vi "PDF Protokoll EPA1065_InterferenceVerification.vi"(8 "error in (no error)":errorcluster caption="Fehler (Eingang, kein Fehler)") -> (0 "error out":errorcluster caption="Fehler (Ausgang)")   [LabVIEW 2020, in "EPA 1065.lvlib" / "Interference verificaton 1065-366.lvlib"]
uses:
  Interference verificaton 1065-366.lvlib
  Visualisierungs Elemente/String - Ausgabefeld.ctl
  ResultTable.ctl
  Sprachverwaltung/FGV Aktion Tabelle zerlegen.ctl
  <vilib>/Utility/miscctls.llb/LVRowAndColumnTypeDef.ctl
  Aktion FGV Interference.ctl
  Seiten/FT-IR/FGV FT-IR Aktionen.ctl
  Aktion Index uebersetzten.ctl
  Seiten/System Einstellungen V2/Aktioen FGV System Konstanten.ctl
  <vilib>/Utility/miscctls.llb/LVPrintingMarginsTypeDef.ctl
  Allgemein/allgemeine Sub-VIs.lvlib
  Seiten/FT-IR/Span/Spanfaktor.lvlib
  Seiten/FT-IR/FT-IR.lvlib
  Sprachverwaltung/Sprachverwaltung.lvlib
  Seiten/System Einstellungen V2/System Einstellungen V2.lvlib
panel:
  out "Grenze in ppm:":sgl=2.0 caption="Limit in ppm:" min=0 format="%#.6g"
  out "[%]":sgl=2.0 caption="Limit:" min=0 format="%#.6g"
  out "LIN Ausgabetabelle":T1
  out "[%]":sgl=120.0 caption="Interference:" min=0 format="%#.6g"
  out "Konzentration Komponente":sgl=120.0 caption="Concentration:" min=0
  out "Komponente:":T2 caption="ppm"
  out "max. Flow Weighted Mean:":T2 caption="%"
  out "Konzentration FlowWeightedMean":sgl=120.0 caption="Concentration:" min=0 format="%#.2f"
  out "Tabelle 3":string[][](table)
  out "Tabelle":string[][](table)
  # "Interference Verification - EPA § 1065.366"
  # "Result"
  # "Analysis"
  # "Interference for Component:"
  # "Expected Flow weighted mean:"
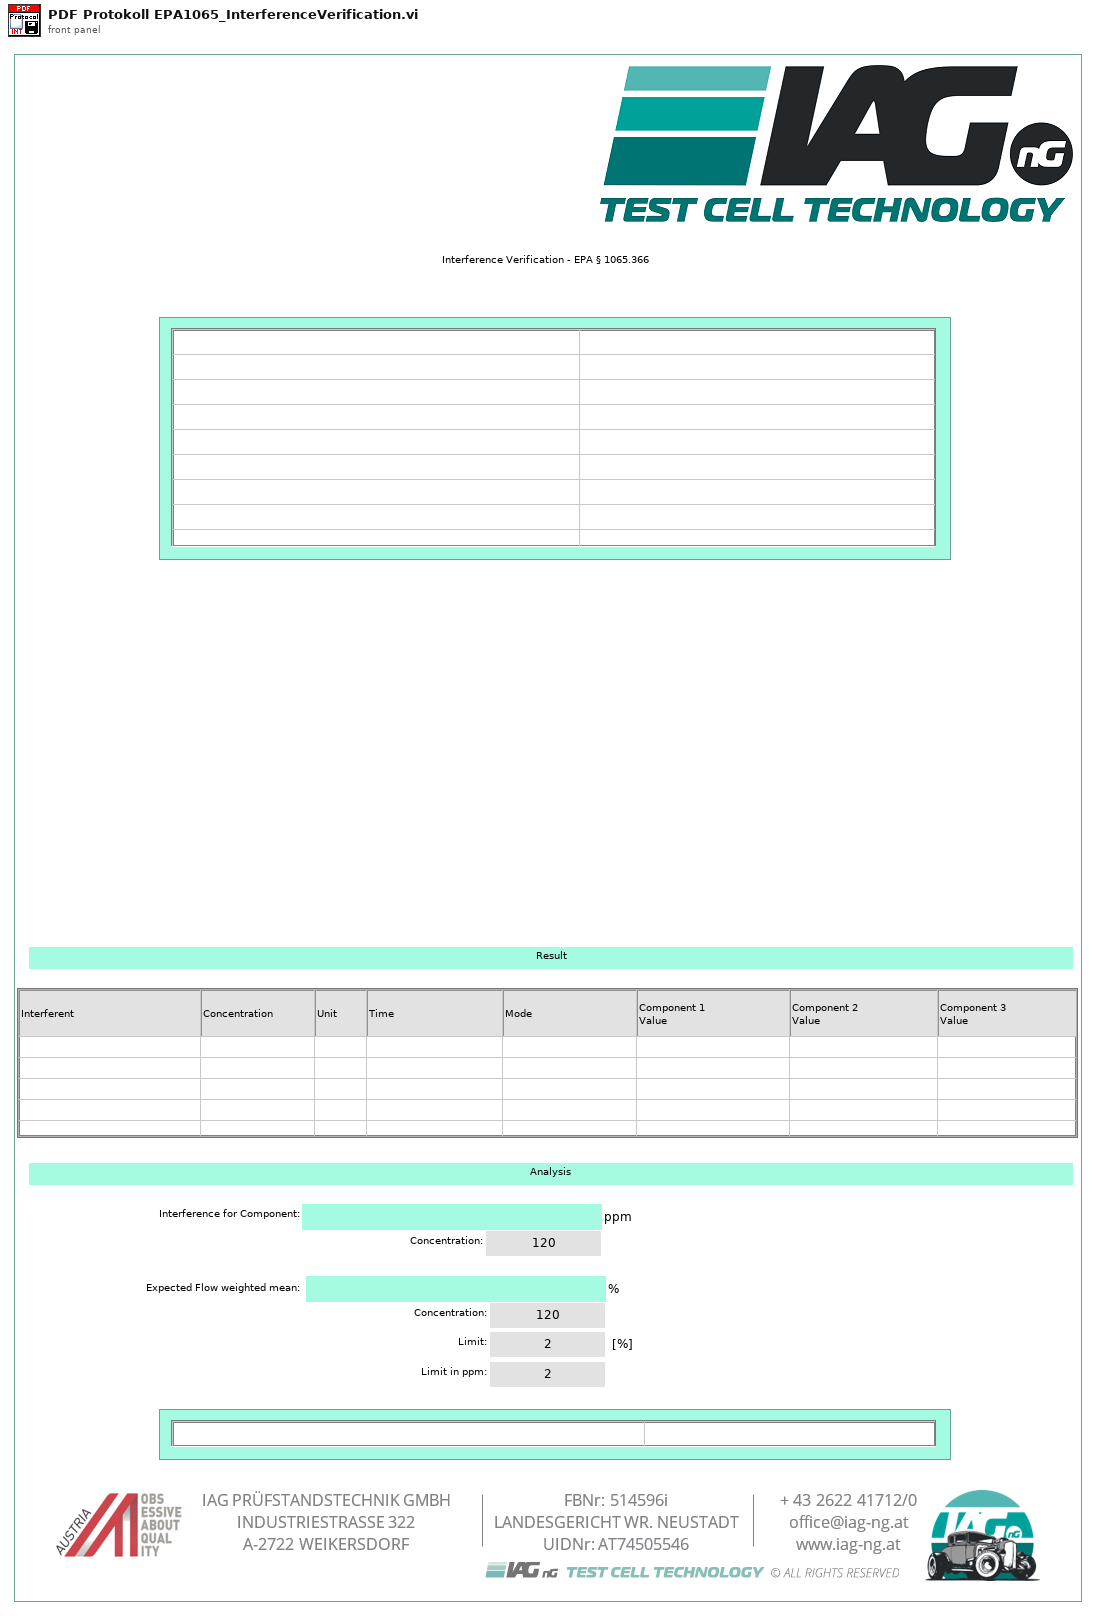
[diagram p1: front panel]
types:
  T1 = typedef "EPA 1065.lvlib/Interference verificaton 1065-366.lvlib/ResultTable.ctl" = string[][]
  T2 = typedef "String - Ausgabefeld.ctl" = string
  T3 = typedef "Sprachverwaltung.lvlib/FGV Aktion Tabelle zerlegen.ctl" = enum16{"laden", "vereinzeln", "speichern"}
  T4 = typedef "System Einstellungen V2.lvlib/Aktioen FGV System Konstanten.ctl" = enum16{"lesen", "laden", "speichern", "Sprache"}
  T5 = typedef "EPA 1065.lvlib/Interference verificaton 1065-366.lvlib/Aktion Index uebersetzten.ctl" = enum16{"lesen", "schreiben", "auswerten"}
  T6 = typedef "FT-IR.lvlib/FGV FT-IR Aktionen.ctl" = enum16{"lesen", "NOG setzen", "NOS setzen", "Initialisieren", "speichern", "ALLES setzen", "FT-IR Spektrum loggen", "Komm Stoppen", "Spektrum LogKonfig"}
  T7 = typedef "EPA 1065.lvlib/Interference verificaton 1065-366.lvlib/Aktion FGV Interference.ctl" = enum16{"Lesen", "TestKonfig", "TestSetting", "Einheiten", "Ergebnis", "Laden", "Tabelle", "Speichern", "löschen"}
  T8 = typedef "LVRowAndColumnTypeDef.ctl" = cluster{"Row":i32, "Column":i32}
  T9 = typedef "LVPrintingMarginsTypeDef.ctl" = cluster{"Top":sgl, "Left":sgl, "Bottom":sgl, "Right":sgl, "Measurement System":enum8{"Inches", "cm"}}
  T10 = enum32{"Portrait", "Landscape", "Rotated Portrait", "Rotated Landscape"}
  T11 = typedef "EPA 1065.lvlib/Interference verificaton 1065-366.lvlib/TestSetting.ctl" = cluster{"Bearbeiter:":string, "Pfad:":path, "Textname:":string, "Analysator":T12}
  T12 = typedef "System Einstellungen V2.lvlib/Analysatoren.ctl" = string
  T13 = typedef "EPA 1065.lvlib/Interference verificaton 1065-366.lvlib/TestKonfig.ctl" = cluster{"CH4:":u16, "Ethane:":u16, "NMHC:":u16, "NMNEHC:":u16, "Komp 1 aktiv:":bool, "Komp 2 aktiv:":bool, "Komp 3 aktiv:":bool, "Komp 4 aktiv:":bool, "Modus":T14, "CG Aufschaltzeit:":dbl, "Interferent 1: CO2":u16, "Interferent 2: H2O":u16, "Interferent 3: CH4":u16, "Interferent 4: C2H6 / C3H8":u16, "Gasflaschen Nr.:":string, "Gasflaschen Nr.: 3":string, "Gasflaschen Nr.: 4":string, "Inter 1 aktiv":bool, "Inter 2 aktiv":bool, "Inter 3 aktiv":bool, "Inter 4 aktiv":bool, "Accuracy":string, "Accuracy 3":string, "Accuracy 4":string, "Konzentration 1:":dbl, "Konzentration 2:":dbl, "Konzentration 3:":dbl, "Konzentration 4:":dbl, "Flow weighted mean 1:":dbl, "Flow weighted mean 2:":dbl, "Flow weighted mean 3:":dbl, "Flow weighted mean 4:":dbl}
  T14 = typedef "EPA 1065.lvlib/Interference verificaton 1065-366.lvlib/Modus.ctl" = u16
  T15 = typedef "EPA 1065.lvlib/Interference verificaton 1065-366.lvlib/Komponenten.ctl" = cluster{"Komponente":T2, "Komponente Index":i32, "Komponente 2":T2, "Komponente Index 2":i32, "Komponente 3":T2, "Komponente Index 3":i32, "Komponente 4":T2, "Komponente Index 4":i32, "Interferent 1":T2, "Interferent Index":i32, "Interferent 2":T2, "Interferent 2 Index":i32, "Interferent 3":T2, "Interferent 3 Index":i32, "Interferent 4":T2, "Interferent 4 Index":i32}
  T16 = cluster{"Modell":string, "ProjektNummer":string, "Software Version":string, "Seriennummer":string}
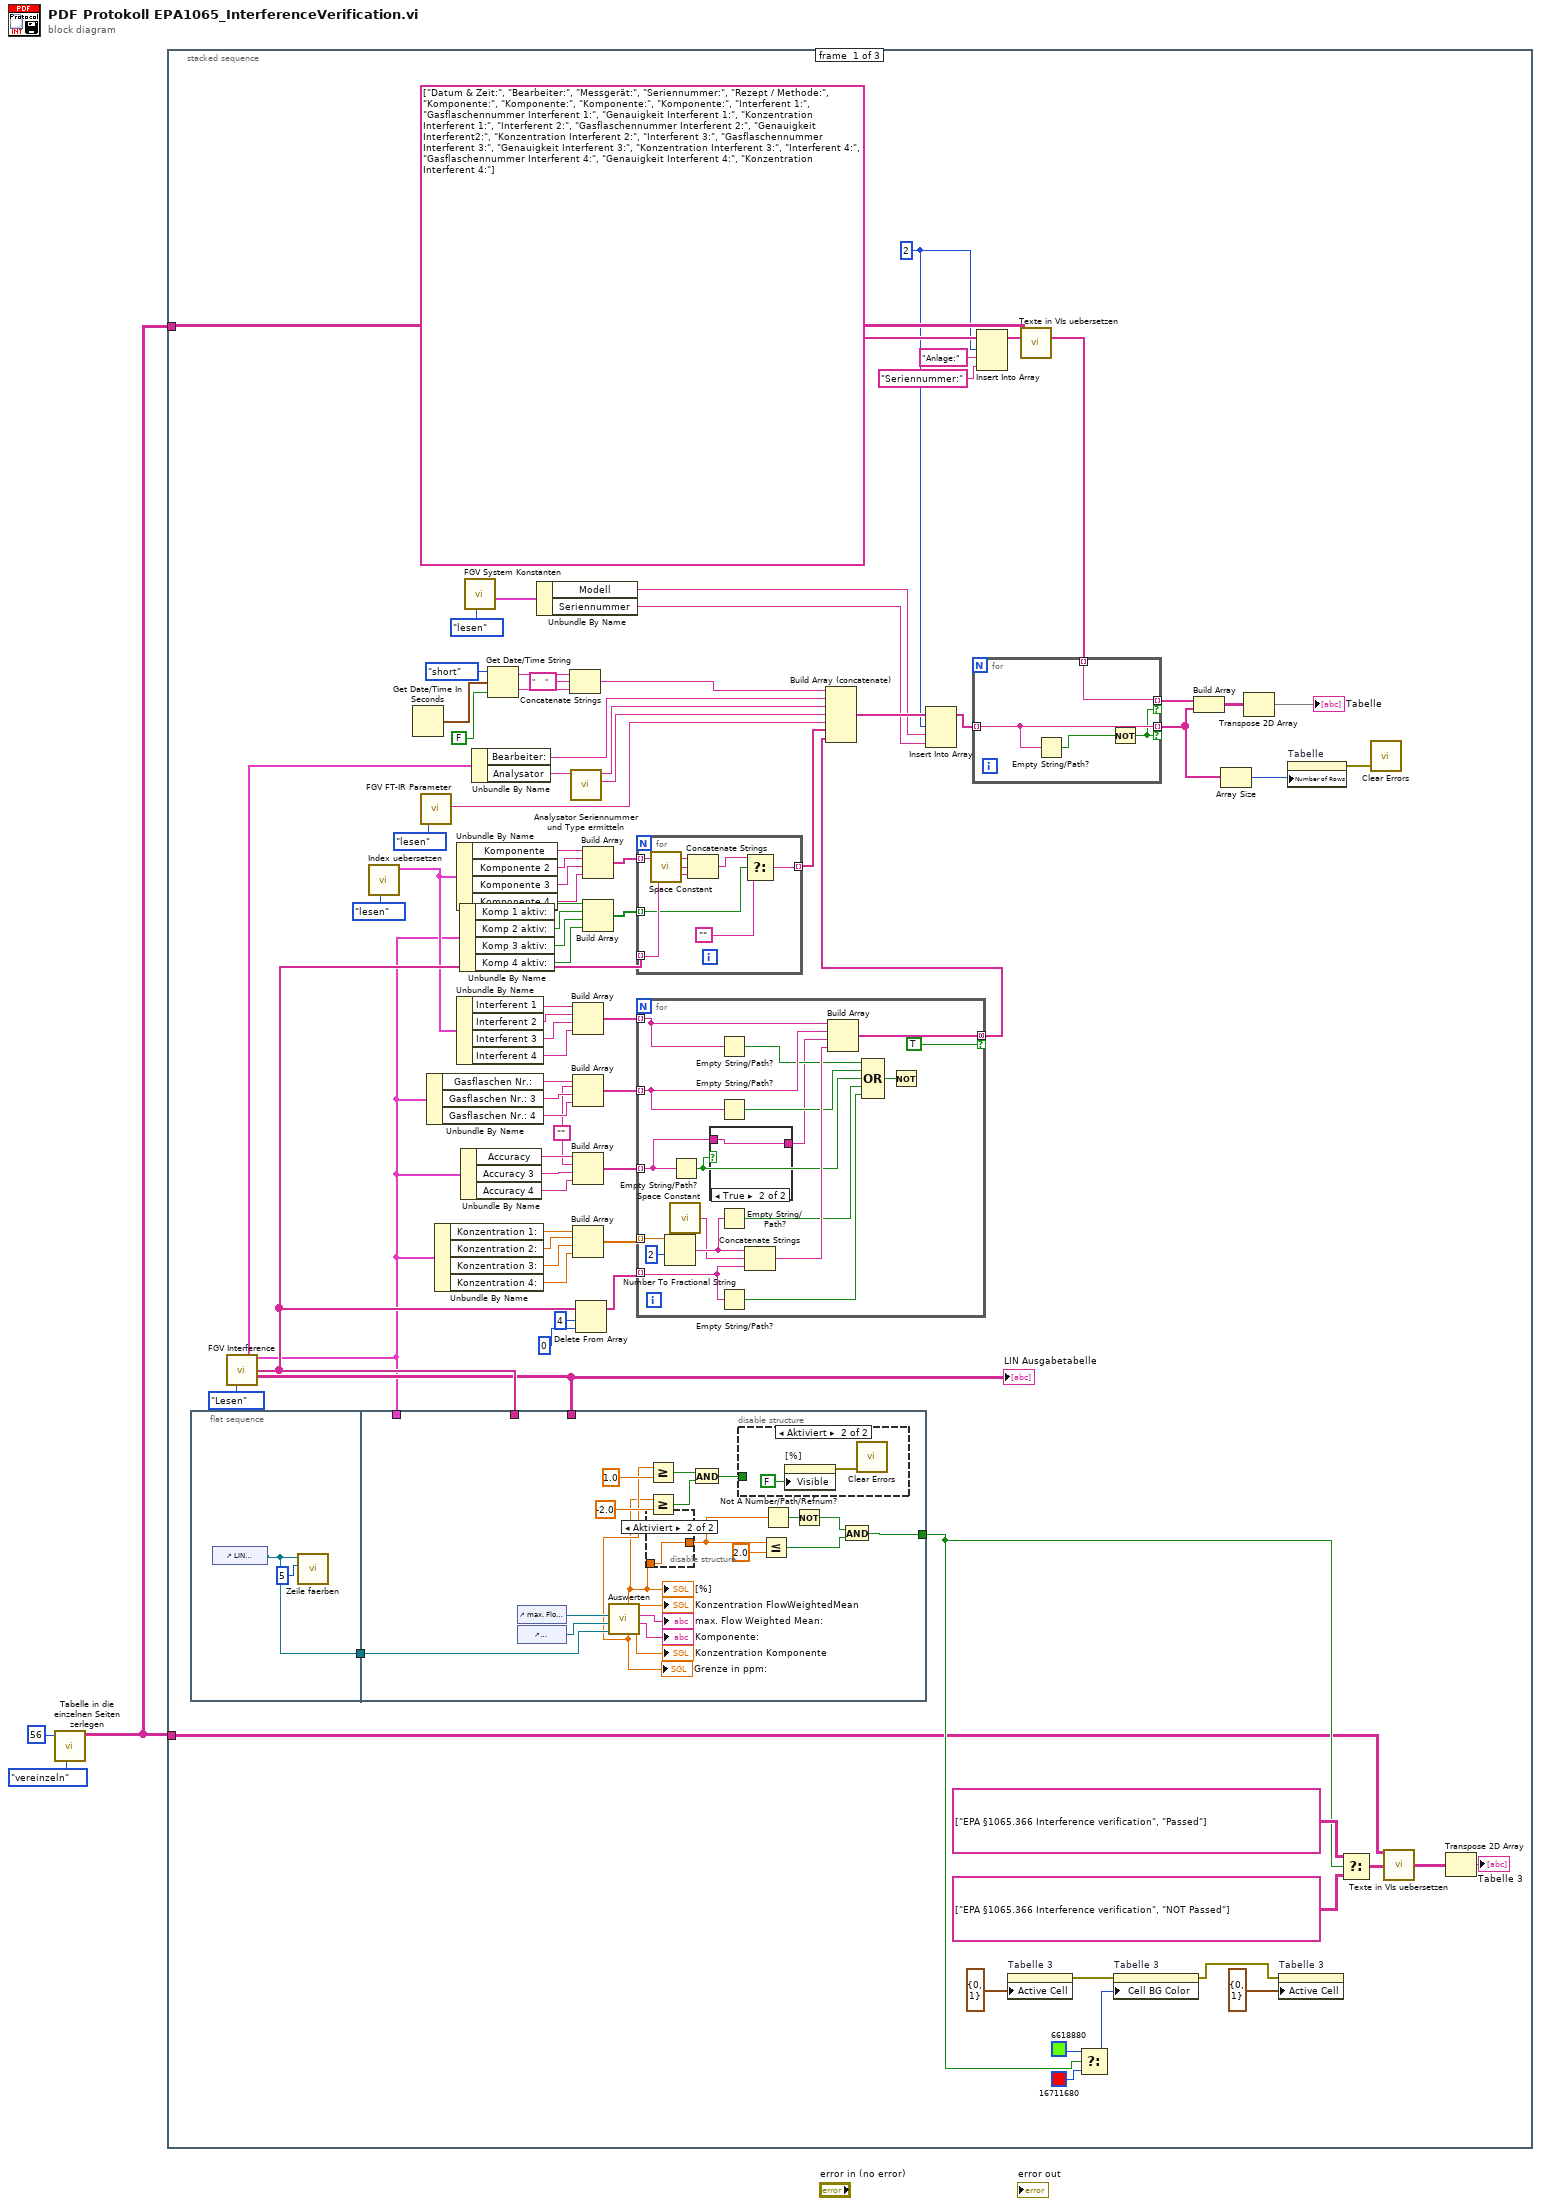
[diagram p0: block diagram]
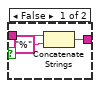
[diagram p2: hidden frame]
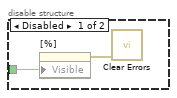
[diagram p3: hidden frame]
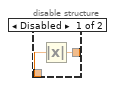
[diagram p4: hidden frame]
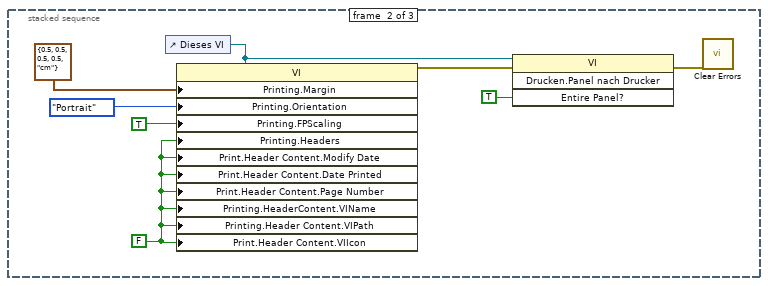
[diagram p5: hidden frame]
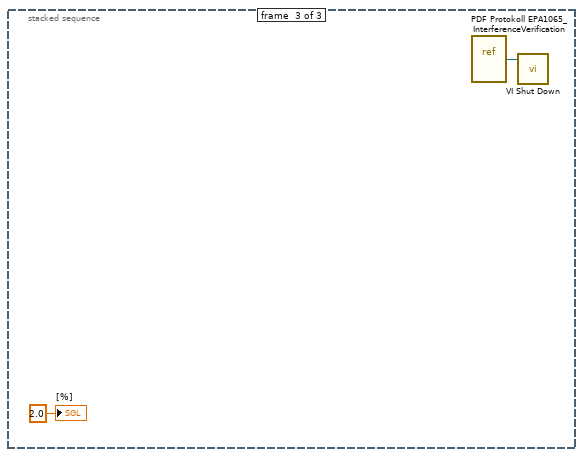
[diagram p6: hidden frame]
diagram:
  n1 = call "Tabelle in die einzelnen Seiten zerlegen.vi"("Aktion"=FGV_Aktion_Tabelle_zerlegen."vereinzeln", "Index (Seite)"=56) -> ("Sprachliste"=w1:string[][])  [unwired: 7 in, 2 out]
  n2 = stacked-sequence {
    tunnel: w1 -> [w24 _ _]
    tunnel: w1 -> [w21 _ _]
    frame #0 {
      w9 = ""
      w10 = 2 ("Index")
      n3 = flat-sequence {
        tunnel: [w125] -> w81
        tunnel: w81 -> [w146]
        tunnel: [w134] -> w80
        tunnel: w51 -> [_]
        tunnel: w27 -> [_]
        tunnel: w20 -> [_]
        frame #0 {
          n4 = control-ref of="LIN Ausgabetabelle"() -> (w125:refnum<vi>)
          n5 = call "Zeile faerben.vi"("Anzahl"=5, "Table (Eingang)"=w125) -> ()  [unwired: 9 in, 1 out]
        }
        frame #1 {
          n6 = control-ref of="max. Flow Weighted Mean:"() -> (w141:refnum<vi>)
          n7 = control-ref of="Komponente:"() -> (w140:refnum<vi>)
          n8 = call "Auswerten.vi"("LIN Ausgabetabelle"=w146, "Komponente:"=w140, "max. Flow Weighted Mean:"=w141) -> ("Konzentration Komponente"=→"Konzentration Komponente":dbl, "Komponente:"=→"Komponente:":T2, "max. Flow Weighted Mean:"=→"max. Flow Weighted Mean:":T2, "Konzentration FlowWeightedMean"=→"Konzentration FlowWeightedMean":dbl, "Limit in ppm"=w129:dbl, "[%]"=w128:dbl)  [unwired: 3 in]
          "[%]" <- w128
          "Grenze in ppm:" <- w129
          n9 = disable-structure shown="Aktiviert" {
            disable-tunnel: w128 -> [w152 w153]
            disable-tunnel: [w151 w153] -> w138
            frame Disabled {
              n10 = Absolute Value(x=w152) -> (abs(x)=w151:dbl)
            }
            frame Enabled {
            }
          }
          n11 = Greater Or Equal?(x=w129, y=1.0) -> (x >= y?=w131:bool)
          n12 = Greater Or Equal?(x=w128, y=-2.0) -> (x >= y?=w130:bool)
          n13 = And(x=w131, y=w130) -> (x .and. y?=w127:bool)
          n14 = disable-structure shown="Aktiviert" {
            disable-tunnel: w127 -> [w148 _]
            frame Disabled {
              n15 = property on="[%]" class="DigWert (strikt)"("Visible"=w148) -> (error out=w147:errorcluster)  [unwired: 2 in, 1 out]
              n16 = call <vilib>:"Clear Errors.vi"("error in (no error)"=w147) -> ()  [unwired: 5 in, 2 out]
            }
            frame Enabled {
              n17 = property on="[%]" class="DigWert (strikt)"("Visible"=FALSE ("Sichtbar")) -> (error out=w150:errorcluster)  [unwired: 2 in, 1 out]
              n18 = call <vilib>:"Clear Errors.vi"("error in (no error)"=w150) -> ()  [unwired: 5 in, 2 out]
            }
          }
          n19 = Less Or Equal?(x=w138, y=2.0) -> (x <= y?=w136:bool)
          n20 = Not A Number/Path/Refnum?(number/path/refnum=w138) -> (NaN/Path/Refnum?=w137:bool)
          n21 = Not(x=w137) -> (.not. x?=w135:bool)
          n22 = And(x=w135, y=w136) -> (x .and. y?=w134:bool)
        }
      }
      n23 = call "FGV Interference.vi"("Aktion FGV Interference"=Aktion_FGV_Interference."Lesen") -> ("TestSetting"=w78:T11, "TestKonfig"=w20:T13, "Êinheiten"=w51:string[], "Tabelle"=w27:T2[][])  [unwired: 9 in, 2 out]
      "LIN Ausgabetabelle" <- w27
      n24 = call "Index uebersetzen.vi"("Aktion"=Aktion_Index_uebersetzten."lesen") -> ("Komponenten"=w45:T15)  [unwired: 9 in, 1 out]
      n25 = Get Date/Time In Seconds() -> (seconds since 1Jan1904=w77:timestamp)
      n26 = call "FGV FT-IR Parameter.vi"("Aktion"=FGV_FT-IR_Aktionen."lesen") -> ("Current Recipe"=w58:string)  [unwired: 11 in, 7 out]
      n27 = Unbundle By Name(w20) -> ("Gasflaschen Nr.:"=w44:string, "Gasflaschen Nr.: 3"=w43:string, "Gasflaschen Nr.: 4"=w42:string)
      n28 = Unbundle By Name(w20) -> ("Konzentration 1:"=w41:dbl, "Konzentration 2:"=w40:dbl, "Konzentration 3:"=w39:dbl, "Konzentration 4:"=w38:dbl)
      n29 = Unbundle By Name(w45) -> ("Komponente"=w69:T2, "Komponente 2"=w68:T2, "Komponente 3"=w67:T2, "Komponente 4"=w8:T2)
      n30 = Unbundle By Name(w45) -> ("Interferent 1"=w49:T2, "Interferent 2"=w48:T2, "Interferent 3"=w47:T2, "Interferent 4"=w46:T2)
      n31 = Unbundle By Name(w20) -> ("Komp 1 aktiv:"=w66:bool, "Komp 2 aktiv:"=w65:bool, "Komp 3 aktiv:"=w64:bool, "Komp 4 aktiv:"=w7:bool)
      n32 = Unbundle By Name(w20) -> ("Accuracy"=w31:string, "Accuracy 3"=w30:string, "Accuracy 4"=w29:string)
      n33 = call "FGV System Konstanten.vi"("Aktionen"=Aktioen_FGV_System_Konstanten."lesen") -> ("Cluster out"=w18:T16)  [unwired: 6 in, 4 out]
      n34 = Unbundle By Name(w78) -> ("Bearbeiter:"=w60:string, "Analysator"=w6:T12)
      n35 = Get Date/Time String(date format (0)=enum16{"short", "long", "abbreviated"}."short" ("Datumsformat (0)"), seconds (now)=w77, want seconds? (F)=FALSE ("Angabe von Sekunden? (F)")) -> (date string=w76:string, time string=w75:string)
      n36 = Unbundle By Name(w18) -> ("Modell"=w14:string, "Seriennummer"=w13:string)
      n37 = Concatenate Strings(w76, "     " ("String"), w75) -> (w61:string)
      n38 = call "Analysator Seriennummer und Type ermitteln.vi"("Analysator"=w6) -> ("Type"=w4:string, "Name für Protokoll"=w5:string)  [unwired: 8 in, 1 out]
      n39 = Build Array(w49, w48, w47, w46) -> (w37:T2[])
      n40 = Build Array(w44, w9, w43, w42) -> (w36:string[])
      n41 = Build Array(w31, w9, w30, w29) -> (w28:string[])
      n42 = Build Array(w41, w40, w39, w38) -> (w35:dbl[])
      n43 = Delete From Array(array=w51, length=4 ("Länge"), index=0 ("Index")) -> (array with subset deleted=w33:string[])  [unwired: 1 out]
      n44 = Build Array(w69, w68, w67, w8) -> (w63:T2[])
      n45 = Build Array(w66, w65, w64, w7) -> (w62:bool[])
      n46 = for {
        tunnel: [w121] -> w59 mode=indexing
        tunnel: w63 -> [w124] mode=indexing
        tunnel: w62 -> [w120] mode=indexing
        tunnel: w51 -> [w123] mode=indexing
        n47 = call <vilib>:"Space Constant.vi"() -> ("String"=w122:string)
        n48 = Concatenate Strings(w124, w122, w123) -> (w119:string)
        n49 = Select(t=w119, s=w120, f="") -> (s? t:f=w121:string)
      }
      n50 = for {
        tunnel: w37 -> [w106] mode=indexing
        tunnel: w36 -> [w105] mode=indexing
        tunnel: w35 -> [w109] mode=indexing
        tunnel: w33 -> [w108] mode=indexing
        tunnel: [w103] -> w32 mode=concatenating if=TRUE
        tunnel: w28 -> [w93] mode=indexing
        n51 = Number To Fractional String(number=w109, precision (6)=i16 2 ("Genauigkeit (6)")) -> (F-format string=w107:string)  [unwired: 2 in]
        n52 = call <vilib>:"Space Constant.vi"() -> ("String"=w97:string)
        n53 = Empty String/Path?(string/path=w93) -> (empty?=w92:bool)
        n54 = case shown="True" w92 {
          tunnel: [w111 w113] -> w96
          tunnel: w93 -> [w110 w113]
          frame False {
            n55 = Concatenate Strings(w110, "%" ("String")) -> (w111:string)
          }
          frame True {
          }
        }
        n56 = Empty String/Path?(string/path=w106) -> (empty?=w102:bool)
        n57 = Empty String/Path?(string/path=w105) -> (empty?=w101:bool)
        n58 = Empty String/Path?(string/path=w107) -> (empty?=w98:bool)
        n59 = Empty String/Path?(string/path=w108) -> (empty?=w100:bool)
        n60 = Concatenate Strings(w107, w97, w108) -> (w104:string)
        n61 = Build Array(w106, w105, w96, w104) -> (w103:T2[])
        n62 = Compound Arithmetic op=OR ("Mehrfacharithmetik")(w102, w101, w92, w98, w100) -> (w99:bool)
        n63 = Not(x=w99) -> ()  [unwired: 1 out]
      }
      n64 = Build Array (concatenate)(w61, w60, w5, w4, w58, w59, w32) -> (w16:T2[])
      n65 = Insert Into Array(array=w16, index=w10, new element #1=w14, new element #2=w13) -> (w15:T2[])
      n66 = Insert Into Array(array=string[] ["Datum & Zeit:", "Bearbeiter:", "Messgerät:", "Seriennummer:", "Rezept / Methode:", "Komponente:", "Komponente:", "Komponente:", "Komponente:", "Interferent 1:", "Gasflaschennummer Interferent 1:", "Genauigkeit Interferent 1:", "Konzentration Interferent 1:", "Interferent 2:", "Gasflaschennummer Interferent 2:", "Genauigkeit Interferent2:", "Konzentration Interferent 2:", "Interferent 3:", "Gasflaschennummer Interferent 3:", "Genauigkeit Interferent 3:", "Konzentration Interferent 3:", "Interferent 4:", "Gasflaschennummer Interferent 4:", "Genauigkeit Interferent 4:", "Konzentration Interferent 4:"], index=w10, new element #1="Anlage:" ("Neues Element/Teil-Array"), new element #2="Seriennummer:" ("Neues Element/Teil-Array")) -> (w17:string[])
      n67 = property on="Tabelle 3" class="Tbl (strikt)"("Active Cell"=T8 {"Row"=0, "Column"=1} ("Aktive Zelle:Aktive Zelle")) -> (error out=w87:errorcluster)  [unwired: 2 in, 1 out]
      n68 = call "Texte in VIs uebersetzen.vi"("Sprachliste"=w21, "String-Array zum Übersetzen"=w17) -> ("String-Array zum Übersetzen"=w22:string[])  [unwired: 9 in, 4 out]
      n69 = for {
        tunnel: w15 -> [w117] mode=indexing
        tunnel: [w117] -> w54 mode=indexing if=w114
        tunnel: [w115] -> w57 mode=indexing if=w114
        tunnel: w22 -> [w115] mode=indexing
        n70 = Empty String/Path?(string/path=w117) -> (empty?=w116:bool)
        n71 = Not(x=w116) -> (.not. x?=w114:bool)
      }
      n72 = Select(t=u32 6618880, s=w80, f=u32 16711680) -> (s? t:f=w88:u32)
      n73 = property on="Tabelle 3" class="Tbl (strikt)"(error in=w87, "Cell BG Color"=w88) -> (error out=w82:errorcluster)  [unwired: 1 in, 1 out]
      n74 = Build Array(w57, w54) -> (w56:T2[][])
      n75 = Array Size(array=w54) -> (size(s)=w53:i32)
      n76 = Transpose 2D Array(2D array=w56) -> (transposed array=→"Tabelle":T2[][])
      n77 = property on="Tabelle 3" class="Tbl (strikt)"(error in=w82, "Active Cell"=T8 {"Row"=0, "Column"=1} ("Aktive Zelle:Aktive Zelle")) -> ()  [unwired: 1 in, 2 out]
      n78 = property on="Tabelle" class="Tbl (strikt)"("Number of Rows"=w53) -> (error out=w52:errorcluster)  [unwired: 2 in, 1 out]
      n79 = Select(t=string[][] [["EPA §1065.366 Interference verification"], ["Passed"]] ("Tabelle 3"), s=w80, f=string[][] [["EPA §1065.366 Interference verification"], ["NOT Passed"]] ("Tabelle 3")) -> (s? t:f=w26:string[][])
      n80 = call <vilib>:"Clear Errors.vi"("error in (no error)"=w52) -> ()  [unwired: 5 in, 2 out]
      n81 = call "Texte in VIs uebersetzen.vi"("Sprachliste"=w24, "2D String-Array zum Übersetzen"=w26) -> ("2D String-Array zum Übersetzen"=w25:string[][])  [unwired: 9 in, 4 out]
      n82 = Transpose 2D Array(2D array=w25) -> (transposed array=→"Tabelle 3":string[][])
    }
    frame #1 {
      w157 = FALSE ("Drucken:Kopfzeilen?")
      n83 = control-ref of="Dieses VI"() -> (w154:refnum<vi>)
      n84 = property class="VI"(reference=w154, "Printing.Margin"=T9 {"Top"=0.5, "Left"=0.5, "Bottom"=0.5, "Right"=0.5, "Measurement System"=enum."cm"} ("Drucken:Ränder"), "Printing.Orientation"=T10."Portrait" ("Drucken:Seitenausrichtung"), "Printing.FPScaling"=TRUE ("Drucken:Frontpanel-Skalierung?"), "Printing.Headers"=w157, "Print.Header Content.Modify Date"=w157, "Print.Header Content.Date Printed"=w157, "Print.Header Content.Page Number"=w157, "Printing.HeaderContent.VIName"=w157, "Printing.Header Content.VIPath"=w157, "Print.Header Content.VIIcon"=w157) -> (error out=w161:errorcluster)  [unwired: 1 in, 1 out]
      n85 = invoke class="VI" method="Drucken.Panel nach Drucker"(reference=w154, error in=w161, "Entire Panel?"=TRUE ("Abschnittskopfzeilen?")) -> (error out=w155:errorcluster)  [unwired: 1 in, 3 out]
      n86 = call <vilib>:"Clear Errors.vi"("error in (no error)"=w155) -> ()  [unwired: 5 in, 2 out]
    }
    frame #2 {
      n87 = vi-ref "PDF Protokoll EPA1065_InterferenceVerification.vi"() -> (w163:refnum<vi>)
      n88 = call "VI Shut Down.vi"("VI Referenz"=w163) -> ()  [unwired: 11 in]
      "[%]" <- sgl 2.0 ("[%]")
    }
  }
